vi "用户鉴权.vi"(10 "news":string, 11 "TCP Network Connection in":refnum<k5>) -> (0 "error out":errorcluster, 3 "TCP Network Connection out":refnum<k5>)   [LabVIEW 2015]
uses:
  Database_util/Ctl/database_Method.ctl
  Database_util/Ctl/DNS.ctl
  Global/SeverGlobal.vi
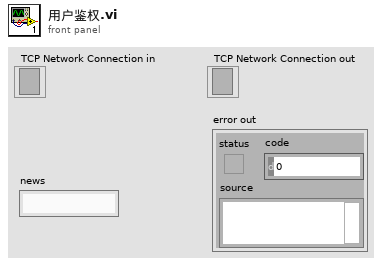
[diagram p1: front panel]
types:
  T1 = typedef "database_Method.ctl" = enum16{"初始化", "查询", "关闭"}
  T2 = typedef "DNS.ctl" = string
  T3 = typedef "响应消息头.ctl" = string
  T4 = cluster{"TCP Ref":refnum<k5>, "Broadcast":refnum<k5>, "TF Ref":refnum<k5>, "IP":string, "port":u16, "userName":string, "passWord":string, "authority":string}[]
  T5 = cluster{"TCP Ref":refnum<k5>, "Broadcast":refnum<k5>, "TF Ref":refnum<k5>, "IP":string, "port":u16, "userName":string, "passWord":string, "authority":string}
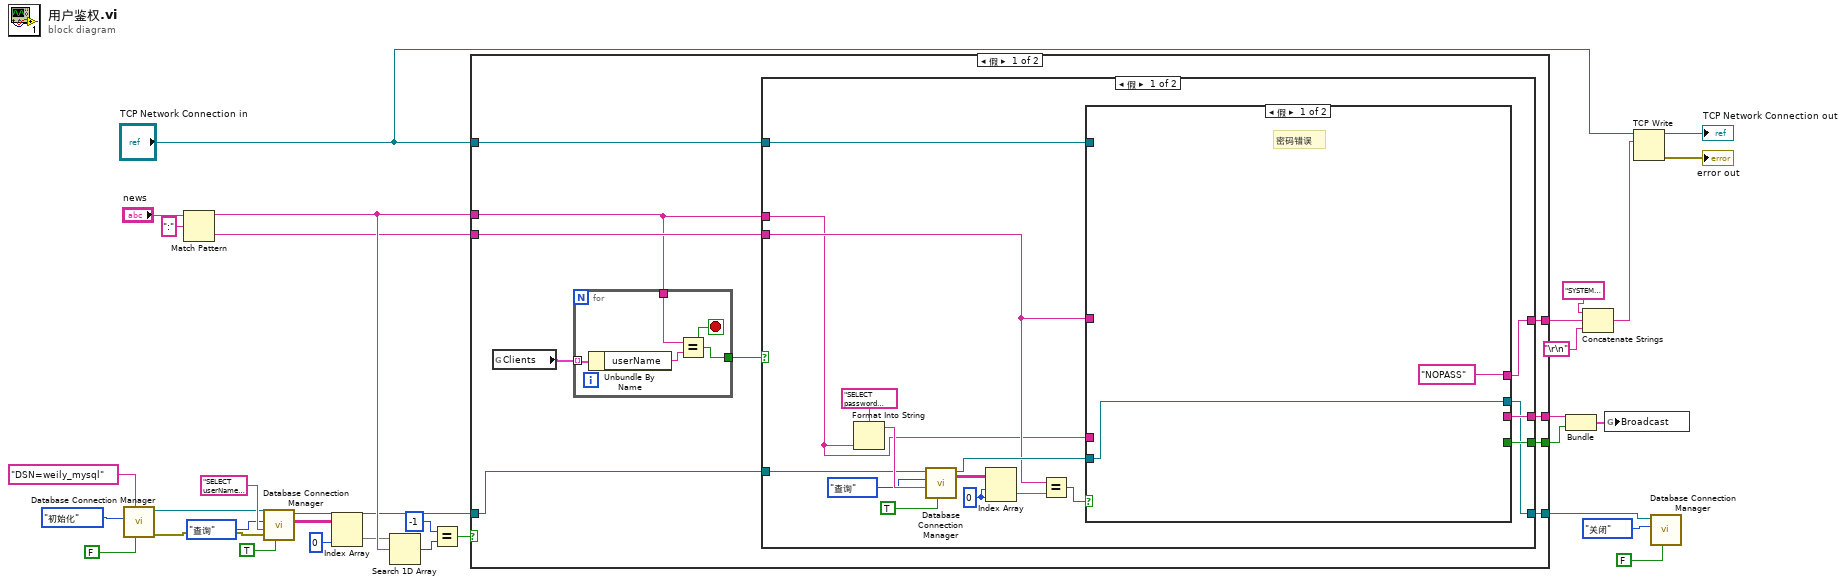
[diagram p0: block diagram]
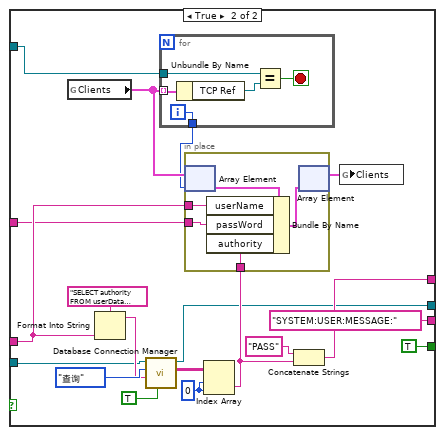
[diagram p2: hidden frame]
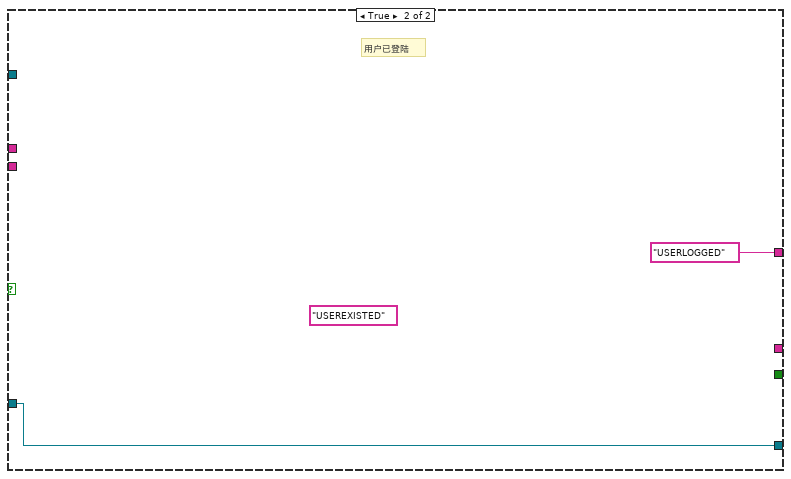
[diagram p3: hidden frame]
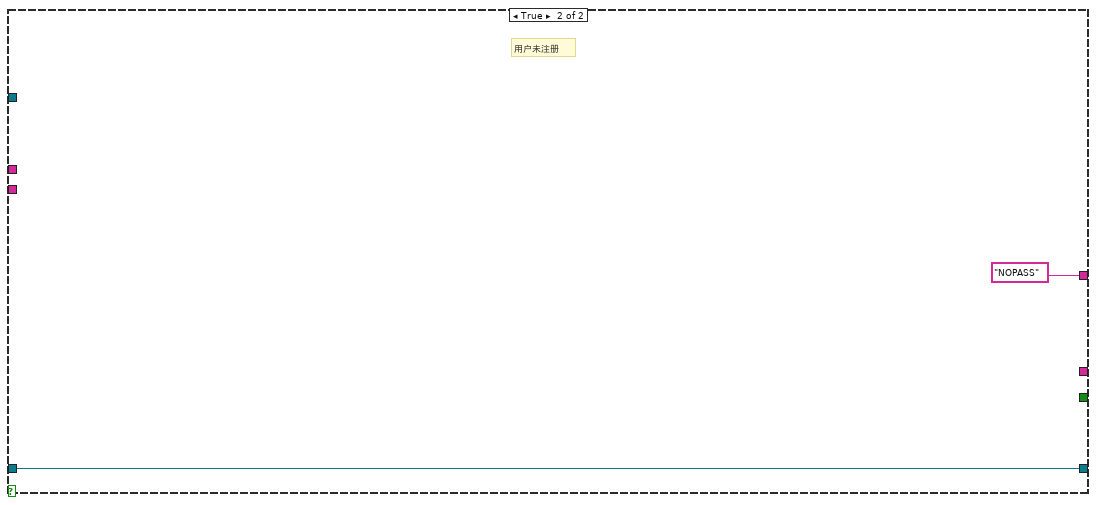
[diagram p4: hidden frame]
diagram:
  n1 = call "Database Connection Manager.vi"("Return Data (T)"=FALSE, "ConnectionString"=T2 "DSN=weily_mysql", "Method"=database_Method."初始化") -> ("error out"=w5:errorcluster, "ADODB._Connection Out"=w4:refnum<k7>)  [unwired: 5 in, 2 out]
  n2 = Match Pattern(string="news", regular expression=":") -> (before substring=w29:string, after substring=w21:string)  [unwired: 1 in, 2 out]
  n3 = call "Database Connection Manager.vi"("Return Data (T)"=TRUE, "error in (no error)"=w5, "Command Text"="SELECT userName FROM userData WHERE isDeled=0" ("SQL"), "Method"=database_Method."查询", "ADODB._Connection In"=w4) -> ("Data"=w15:string[][], "ADODB._Connection Out"=w20:refnum<k7>)  [unwired: 3 in, 2 out]
  n4 = Index Array(array=w15, index (col)=0 ("disabled index (col)")) -> (element=w16:string[])  [unwired: 1 in]
  n5 = Search 1D Array(1D array=w16, element=w29) -> (index of element=w18:i32)  [unwired: 1 in]
  n6 = Equal?(x=-1 ("y"), y=w18) -> (x = y?=w19:bool)
  n7 = case shown="假" w19 {
    tunnel: w20 -> [w38 w97]
    tunnel: [w42 "NOPASS"] -> w22
    tunnel: "TCP Network Connection in" -> [w41 _]
    tunnel: w21 -> [w40 _]
    tunnel: w29 -> [w37 _]
    tunnel: [w35 _] -> w31
    tunnel: [w34 _] -> w32
    tunnel: [w33 w97] -> w1
    frame False {
      n8 = global read "SeverGlobal.vi" "Clients"() -> (w39:T4)
      n9 = for {
        tunnel: w39 -> [w46] mode=indexing
        tunnel: w37 -> [w44]
        tunnel: [w43] -> w36
        stop <- w43 stop-if-true
        n10 = Unbundle By Name(w46) -> ("userName"=w45:string)
        n11 = Equal?(x=w44, y=w45) -> (x = y?=w43:bool)
      }
      n12 = case shown="假" w36 {
        tunnel: [w54 "USERLOGGED" ("element")] -> w42
        tunnel: w38 -> [w56 w95]
        tunnel: w41 -> [w52 _]
        tunnel: w40 -> [w51 _]
        tunnel: w37 -> [w50 _]
        tunnel: [w49 _] -> w35
        tunnel: [w48 _] -> w34
        tunnel: [w47 w95] -> w33
        frame False {
          w63 = 0 ("disabled index (col)")
          n13 = Format Into String(format string="SELECT password FROM userData WHERE isDeled=0 AND userName='%s'" ("SQL"), w50) -> (resulting string=w60:string)  [unwired: 2 in, 1 out]
          n14 = call "Database Connection Manager.vi"("Return Data (T)"=TRUE, "Command Text"=w60, "Method"=database_Method."查询", "ADODB._Connection In"=w56) -> ("Data"=w61:string[][], "ADODB._Connection Out"=w53:refnum<k7>)  [unwired: 4 in, 2 out]
          n15 = Index Array(array=w61, index (row)=w63, index (col)=w63) -> (element=w62:string)
          n16 = Equal?(x=w51, y=w62) -> (x = y?=w55:bool)
          n17 = case shown="假" w55 {
            tunnel: ["NOPASS" w76] -> w54
            tunnel: w53 -> [w64 w80]
            tunnel: w50 -> [_ w71]
            tunnel: w52 -> [_ w75]
            tunnel: w51 -> [_ w70]
            tunnel: [_ "SYSTEM:USER:MESSAGE:"] -> w49
            tunnel: [_ TRUE ("Return Data (T)")] -> w48
            tunnel: [w64 w66] -> w47
            frame False {
              # "密码错误"
            }
            frame True {
              w79 = 0 ("disabled index (col)")
              n18 = global read "SeverGlobal.vi" "Clients"() -> (w74:T4)
              n19 = Format Into String(format string="SELECT authority FROM userData WHERE isDeled=0 AND userName='%s'" ("SQL"), w71) -> (resulting string=w81:string)  [unwired: 2 in, 1 out]
              n20 = call "Database Connection Manager.vi"("Return Data (T)"=TRUE, "Command Text"=w81, "Method"=database_Method."查询", "ADODB._Connection In"=w80) -> ("Data"=w78:string[][], "ADODB._Connection Out"=w66:refnum<k7>)  [unwired: 4 in, 2 out]
              n21 = for {
                tunnel: w74 -> [w94] mode=indexing
                tunnel: w75 -> [w93]
                tunnel: [w90] -> w73
                i -> [w90]
                stop <- w91 stop-if-true
                n22 = Unbundle By Name(w94) -> ("TCP Ref"=w92:refnum<k5>)
                n23 = Equal?(x=w93, y=w92) -> (x = y?=w91:bool)
              }
              n24 = Index Array(array=w78, index (row)=w79, index (col)=w79) -> (element=w69:string)
              n25 = in-place {
                in-place-border: w71 -> [w87]
                in-place-border: w70 -> [w86]
                in-place-border: w69 -> [w85]
                n26 = in-place-array #1(w74, w73) -> (w89:T5)
                n27 = Bundle By Name(cluster=w89, "userName"=w87, "passWord"=w86, "authority"=w85) -> (w88:T5)
                n28 = in-place-array #1(w88) -> (w72:T4)  [unwired: 1 out]
              }
              n29 = Concatenate Strings("PASS", w69) -> (w76:string)
              n30 = global write "SeverGlobal.vi" "Clients"(w72) -> ()
            }
          }
        }
        frame True {
          (unwired) "USEREXISTED" ("element")
          # "用户已登陆"
        }
      }
    }
    frame True {
      # "用户未注册"
    }
  }
  n31 = Bundle(w31, "Return Data (T)"=w32) -> (w30:cluster{string, "Return Data (T)":bool})  [unwired: 1 in]
  n32 = Concatenate Strings(T3 "SYSTEM:RELOGIN:" ("Combo Box"), w22, "\r\n") -> (w24:string)
  n33 = global write "SeverGlobal.vi" "Broadcast"(w30) -> ()
  n34 = TCP Write(connection ID="TCP Network Connection in", data in=w24) -> (connection ID out=→"TCP Network Connection out":refnum<k5>, error out=→"error out":errorcluster)  [unwired: 2 in, 1 out]
  n35 = call "Database Connection Manager.vi"("Return Data (T)"=FALSE, "Method"=database_Method."关闭", "ADODB._Connection In"=w1) -> ()  [unwired: 5 in, 4 out]
